vi "absdifference.vi"() -> ()   [LabVIEW 2021]
uses:
  <vilib>/vision/NI_Vision_Development_Module.lvlib
panel:
  in  "stop":bool
  out "Image Dst Out 2":T1(plugin-control)
  in  "Constant":dbl=1.0 format="%.2f"
  out "error out":errorcluster
  out "Image Dst Out":T1(plugin-control)
  in  "File Path 2":path
  in  "File Path":path
  in  "error in":errorcluster
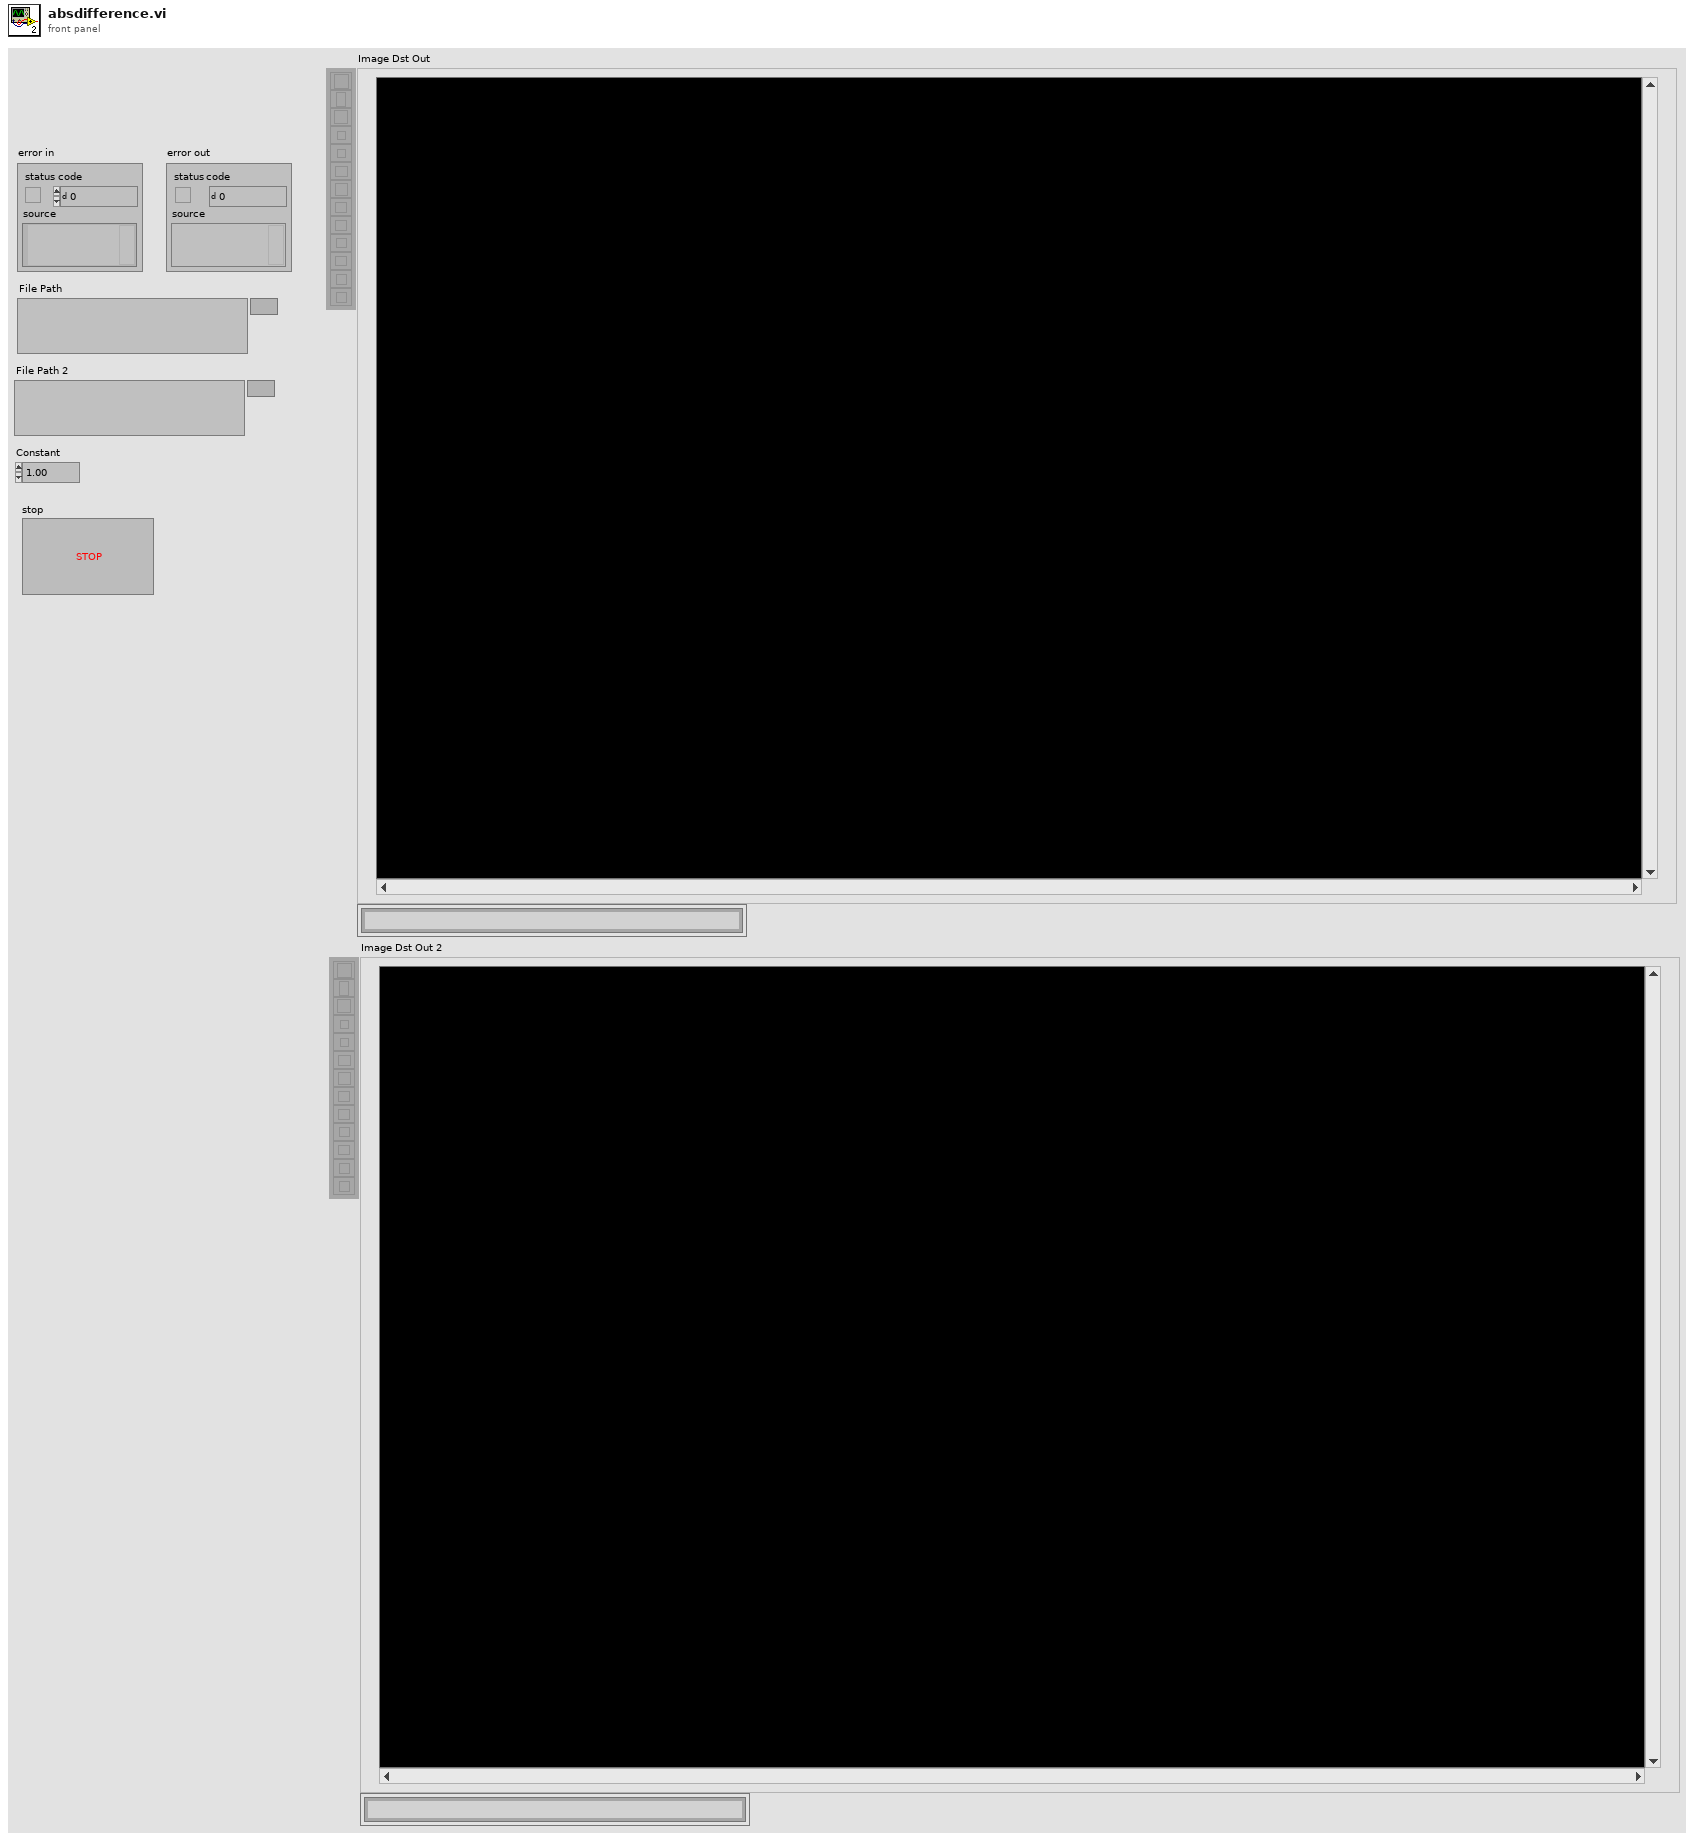
[diagram p1: front panel]
types:
  T1 = typedef "IMAQ Image.ctl" = refnum<image>
  T2 = typedef "Image Type" = u32
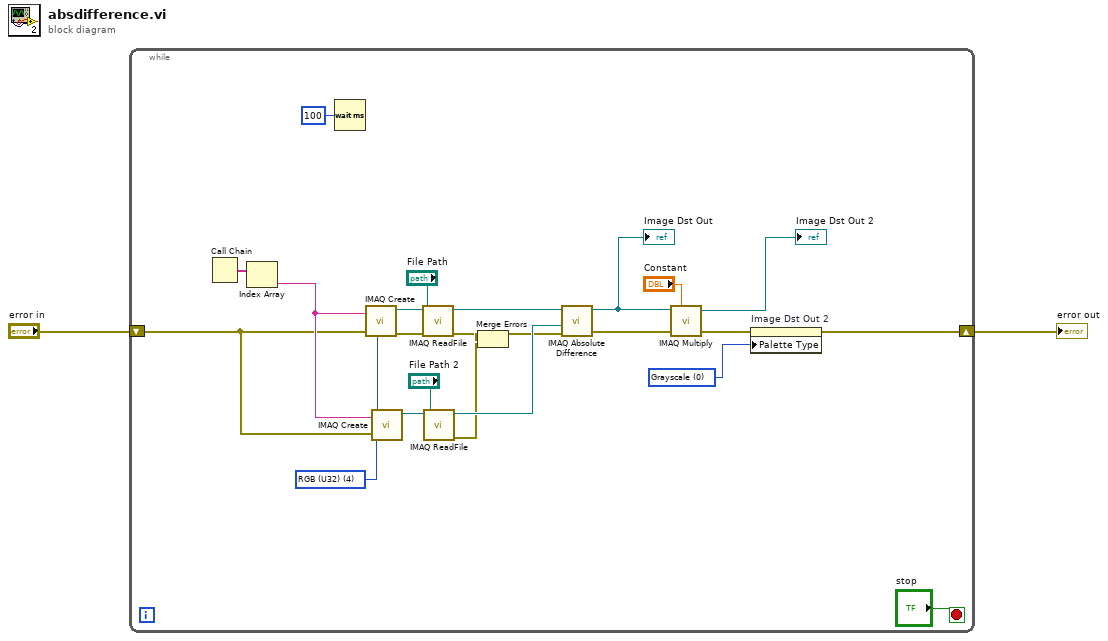
[diagram p0: block diagram]
diagram:
  n1 = while {
    shift-right: [w6] -> w1
    shift-left: "error in" -> [w18]
    stop <- "stop" stop-if-true
    w5 = u32 0 items=["Grayscale", "Binary", "Gradient", "Rainbow", "Temperature", "User Defined", "Binary 16 Bit", "Gradient 16 Bit", "Rainbow 16 Bit", "Temperature 16 Bit", "User Defined 16 Bit"] ("Palette Type")
    w17 = T2 4 items=["Grayscale (U8)", "Grayscale (I16)", "Grayscale (SGL)", "Complex (CSG)", "RGB (U32)", "HSL (U32)", "RGB (U64)", "Grayscale (U16)"] ("Image Type")
    n2 = Call Chain() -> (call chain=w23:string[])
    n3 = Index Array(array=w23) -> (element=w19:string)  [unwired: 1 in]
    n4 = Wait (ms)(milliseconds to wait=u32 100) -> ()  [unwired: 1 out]
    n5 = call "IMAQ Create"("Image Name"=w19, "Image Type"=w17, "error in (no error)"=w18) -> ("New Image"=w25:T1, "error out"=w24:errorcluster)  [unwired: 1 in, 1 out]
    n6 = call "IMAQ Create"("Image Name"=w19, "Image Type"=w17, "error in (no error)"=w18) -> ("New Image"=w20:T1)  [unwired: 1 in, 2 out]
    n7 = call "IMAQ ReadFile"("File Path"="File Path", "error in (no error)"=w24, "Image"=w25) -> ("error out"=w13:errorcluster, "Image Out"=w21:T1)  [unwired: 2 in, 5 out]
    n8 = call "IMAQ ReadFile"("File Path"="File Path 2", "Image"=w20) -> ("error out"=w12:errorcluster, "Image Out"=w15:T1)  [unwired: 3 in, 5 out]
    n9 = Merge Errors(w13, w12) -> (w14:errorcluster)
    n10 = call "IMAQ Absolute Difference"("Image Src A"=w21, "Image Src B"=w15, "error in (no error)"=w14) -> ("Image Dst Out"=w11:T1, "error out"=w10:errorcluster)  [unwired: 2 in, 2 out]
    "Image Dst Out" <- w11
    n11 = call "IMAQ Multiply"("Image Src A"=w11, "Constant"="Constant", "error in (no error)"=w10) -> ("Image Dst Out"=→"Image Dst Out 2":T1, "error out"=w7:errorcluster)  [unwired: 2 in, 2 out]
    n12 = property on="Image Dst Out 2" class="ImageControl"(error in=w7, "Palette Type"=w5) -> (error out=w6:errorcluster)  [unwired: 1 in, 1 out]
  }
  "error out" <- w1
